vi "例4-19（2）.vi"() -> ()   [LabVIEW 2019]
panel:
  in  "停止":bool
  out "数值显示":dbl(knob) scale=0.0..10.0
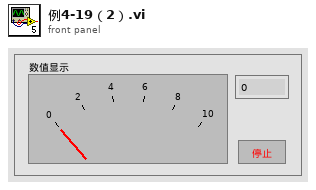
[diagram p1: front panel]
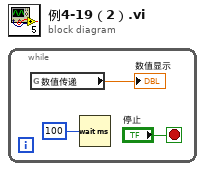
[diagram p0: block diagram]
diagram:
  n1 = while {
    stop <- "停止" stop-if-true
    n2 = global read "例4-19（全局变量）.vi" "数值传递"() -> (→"数值显示":dbl)
    n3 = Wait (ms)(milliseconds to wait=100) -> ()  [unwired: 1 out]
  }
